vi "EKF_Test.vi"() -> ()   [LabVIEW 2019]
uses:
  <vilib>/ptbypt/NI_PtbyPt.lvlib
panel:
  out "delta S":dbl[](array[numeric])=[2.001337986602958, 1.997084886991216]
  out "XY Graph":cluster{dbl[], dbl[]}[](graph)
  in  "w_L":dbl=0.001
  in  "w_R":dbl=0.002
  in  "stop":bool
  in  "milliseconds to wait":u32=10
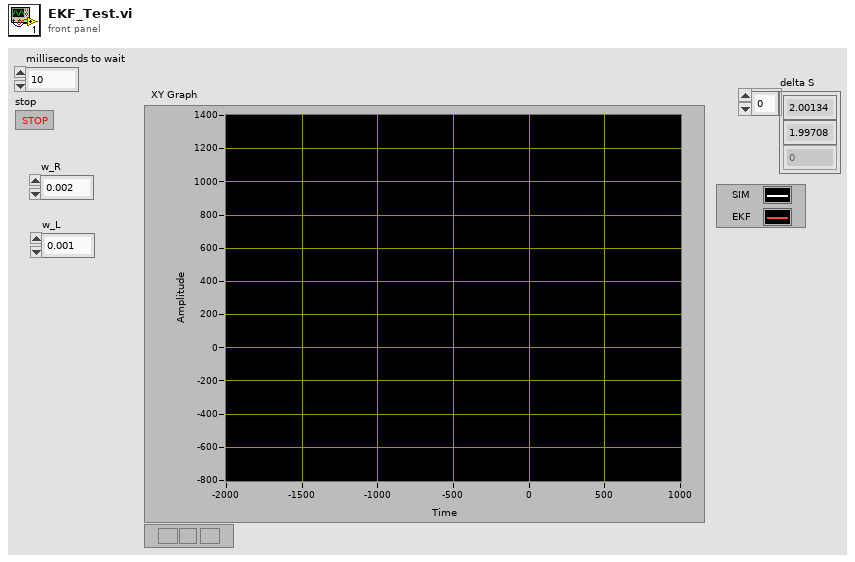
[diagram p1: front panel]
types:
  T1 = typedef "coordinate.ctl" = dbl[]
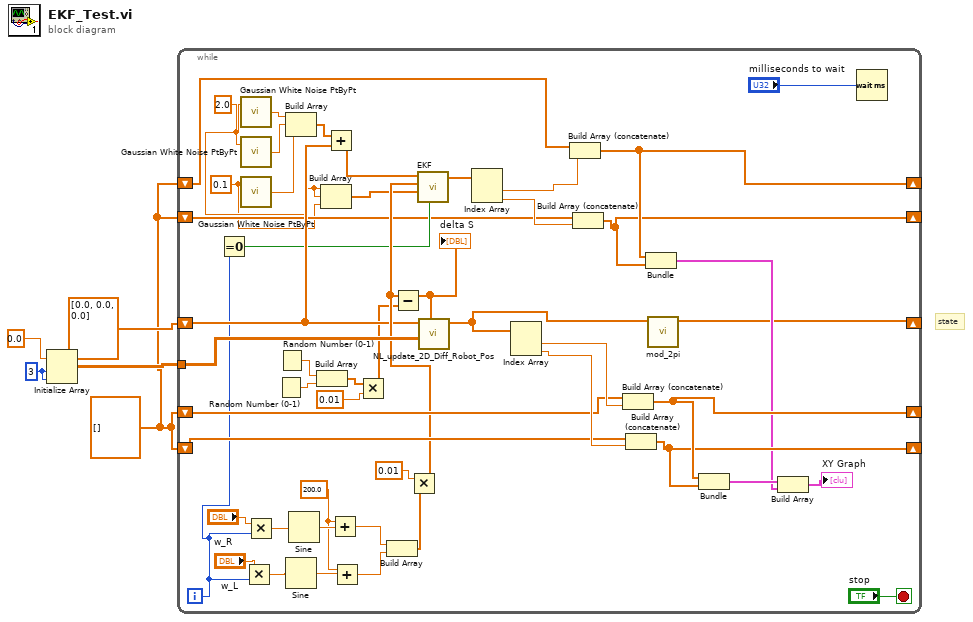
[diagram p0: block diagram]
diagram:
  w1 = dbl[] []
  w4 = 3 ("dimension size")
  # "state"
  n1 = Initialize Array(0.0, w4, w4) -> (w2:dbl[][])
  n2 = while {
    shift-right: [w20] -> _
    shift-left: dbl[] [0.0, 0.0, 0.0] -> [w33]
    tunnel: w2 -> [w47]
    shift-right: [w39] -> _
    shift-left: w1 -> [w41]
    shift-right: [w38] -> _
    shift-left: w1 -> [w40]
    shift-right: [w23] -> _
    shift-left: w1 -> [w24]
    shift-right: [w22] -> _
    shift-left: w1 -> [w27]
    i -> [w32]
    stop <- "stop" stop-if-true
    w9 = 2.0 ("standard deviation")
    w6 = 0.1 ("standard deviation")
    w35 = 200.0 ("x")
    n3 = Equal To 0?(x=w32) -> (x = 0?=w31:bool)
    n4 = call <vilib>:"Gaussian White Noise PtByPt.vi"("standard deviation"=w9) -> ("Gaussian white noise"=w11:dbl)  [unwired: 2 in]
    n5 = call <vilib>:"Gaussian White Noise PtByPt.vi"("standard deviation"=w9) -> ("Gaussian white noise"=w10:dbl)  [unwired: 2 in]
    n6 = call <vilib>:"Gaussian White Noise PtByPt.vi"("standard deviation"=w6) -> ("Gaussian white noise"=w8:dbl)  [unwired: 2 in]
    n7 = Multiply(x="w_L", y=w32) -> (x*y=w50:dbl)
    n8 = Multiply(x="w_R", y=w32) -> (x*y=w51:dbl)
    n9 = Random Number (0-1)() -> (number: 0 to 1=w18:dbl)
    n10 = Random Number (0-1)() -> (number: 0 to 1=w19:dbl)
    n11 = Build Array(w11, w10, w8) -> (w12:dbl[])
    n12 = Sine(x=w50) -> (sin(x)=w48:dbl)
    n13 = Sine(x=w51) -> (sin(x)=w49:dbl)
    n14 = Build Array(w19, w18) -> (w17:dbl[])
    n15 = Build Array(w9, w9, w6) -> (w7:dbl[])
    n16 = Add(x=w12, y=w33) -> (x+y=w13:T1)
    n17 = Add(x=w35, y=w49) -> (x+y=w45:dbl)
    n18 = Add(x=w35, y=w48) -> (x+y=w46:dbl)
    n19 = Multiply(x=w17, y=0.01) -> (x*y=w14:dbl[])
    n20 = Build Array(w45, w46) -> (w44:dbl[])
    n21 = Multiply(x=0.01, y=w44) -> (x*y=w34:dbl[])
    n22 = Subtract(x=w34, y=w14) -> (x-y=w15:dbl[])
    "delta S" <- w15
    n23 = call "EKF.vi"("init"=w31, "Messrausch"=w7, "input"=w34, "Measurements"=w13) -> ("act filtered coord"=w28:T1)  [unwired: 7 in]
    n24 = call "NL_update_2D_Diff_Robot_Pos.vi"("Input Delta s"=w15, "Fk"=w47, "state k"=w33) -> ("state k+1"=w21:T1)  [unwired: 7 in, 1 out]
    n25 = Index Array(array=w28) -> (element #1=w30:dbl, element #2=w29:dbl)  [unwired: 2 in]
    n26 = Index Array(array=w21) -> (element #1=w43:dbl, element #2=w42:dbl)  [unwired: 2 in]
    n27 = Build Array (concatenate)(w24, w30) -> (w23:dbl[])
    n28 = Build Array (concatenate)(w27, w29) -> (w22:dbl[])
    n29 = Build Array (concatenate)(w41, w43) -> (w39:dbl[])
    n30 = Build Array (concatenate)(w40, w42) -> (w38:dbl[])
    n31 = Bundle(w23, w22) -> (w25:cluster{dbl[], dbl[]})  [unwired: 1 in]
    n32 = call "mod_2pi.vi"("state k+1"=w21) -> ("state_mod2pi"=w20:T1)  [unwired: 10 in]
    n33 = Bundle(w39, w38) -> (w37:cluster{dbl[], dbl[]})  [unwired: 1 in]
    n34 = Build Array(w37, w25) -> (→"XY Graph":cluster{dbl[], dbl[]}[])
    n35 = Wait (ms)(milliseconds to wait="milliseconds to wait") -> ()  [unwired: 1 out]
  }
